vi "RPI2 Enable I2C.vi"(8 "Error In":errorcluster, 11 "Install LV Data":T1={"SSH Session"=refnum, "Status Log"="", "Detailed Log"="", "Credentials"={"Hostname or IP"="192.168.7.2", "Username"="root", "Password"=""}, "Target Info"={"OS Version"="", "CPU"="", "Systemd Version"="", "Internet Access"=FALSE, "Device Type"="", "LV Installed Ver"="", "LV Available Ver"="", "LV Upgrade Available"=FALSE, "Hostname"="", "NIC Info"=[]}, "Reboot Required?"=FALSE}) -> (0 "Error Out":errorcluster, 1 "Log":string, 3 "Install LV Data":T1={"SSH Session"=refnum, "Status Log"="", "Detailed Log"="", "Credentials"={"Hostname or IP"="192.168.7.2", "Username"="root", "Password"=""}, "Target Info"={"OS Version"="", "CPU"="", "Systemd Version"="", "Internet Access"=FALSE, "Device Type"="", "LV Installed Ver"="", "LV Available Ver"="", "LV Upgrade Available"=FALSE, "Hostname"="", "NIC Info"=[]}, "Reboot Required?"=FALSE})   [LabVIEW 2019, in "LMH-LINX.lvlib"]
uses:
  <vilib>/MakerHub/LINX/LMH-LINX.lvlib
  <vilib>/MakerHub/LINX/Private/Utilties/Target Management/Install LV Data.ctl
  <vilib>/MakerHub/LINX/Private/Utilties/Target Management/Target Info.ctl
  <vilib>/MakerHub/LINX/Private/Utilties/Target Management/NIC Info.ctl
  <vilib>/MakerHub/LINX/Private/Utilties/Target Management/NIC Mode.ctl
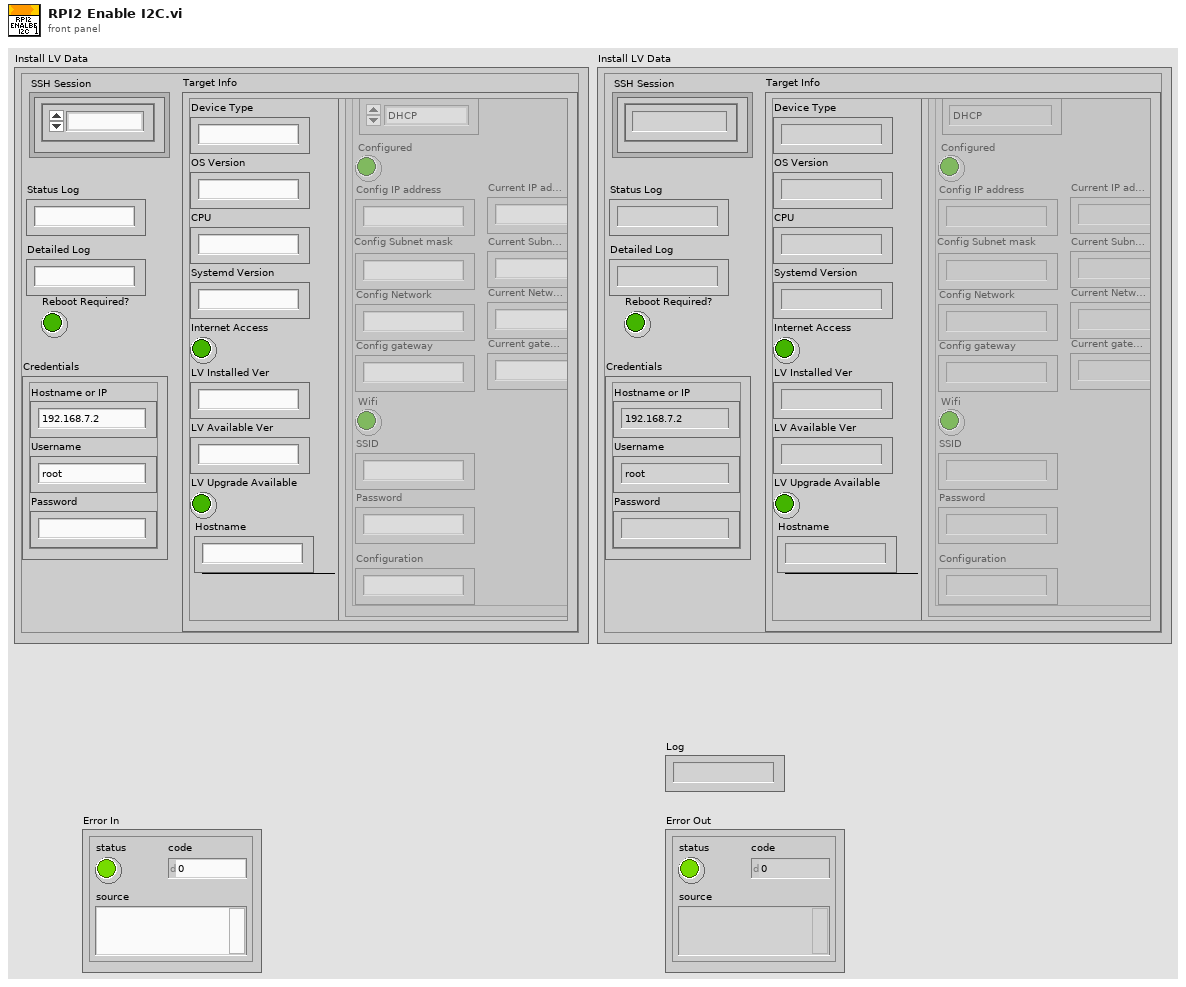
[diagram p1: front panel]
types:
  T1 = typedef "LMH-LINX.lvlib/Install LV Data.ctl" = cluster{"SSH Session":refnum<k1>, "Status Log":string, "Detailed Log":string, "Credentials":cluster{"Hostname or IP":string, "Username":string, "Password":string}, "Target Info":T2, "Reboot Required?":bool}
  T2 = typedef "LMH-LINX.lvlib/Target Info.ctl" = cluster{"OS Version":string, "CPU":string, "Systemd Version":string, "Internet Access":bool, "Device Type":string, "LV Installed Ver":string, "LV Available Ver":string, "LV Upgrade Available":bool, "Hostname":string, "NIC Info":T3[]}
  T3 = typedef "LMH-LINX.lvlib/NIC Info.ctl" = cluster{"Name":string, "NIC Mode":T4, "Configured":bool, "Config IP address":string, "Config Subnet mask":string, "Config Network":string, "Config gateway":string, "Wifi":bool, "SSID":string, "Password":string, "Configuration":string, "Current IP address":string, "Current Subnet mask":string, "Current gateway":string, "Current Network":string}
  T4 = typedef "LMH-LINX.lvlib/NIC Mode.ctl" = enum16{"DHCP", "Static", "Loopback"}
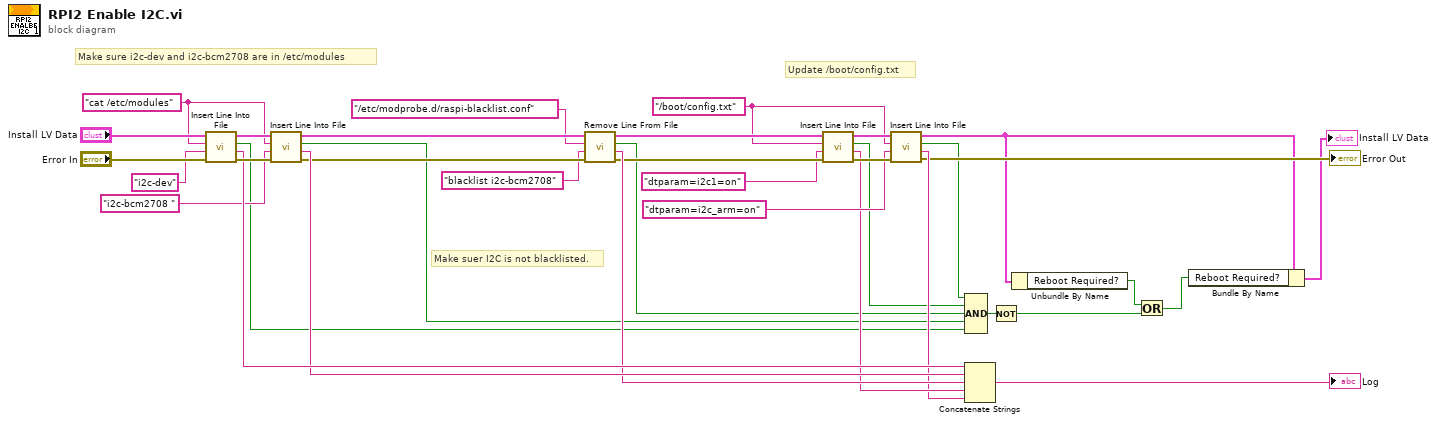
[diagram p0: block diagram]
diagram:
  w15 = "/boot/config.txt"
  w27 = "cat /etc/modules" ("File Path")
  # "Update /boot/config.txt"
  # "Make suer I2C is not blacklisted."
  # "Make sure i2c-dev and i2c-bcm2708 are in /etc/modules"
  n1 = call <vilib>:"Insert Line Into File.vi"("Error In"="Error In", "Line"="i2c-dev" ("File Path"), "File Path"=w27, "Install LV Data"="Install LV Data") -> ("Error Out"=w33:errorcluster, "Log"=w32:string, "Line Alredy Present?"=w7:bool, "Install LV Data"=w34:T1)  [unwired: 4 in]
  n2 = call <vilib>:"Insert Line Into File.vi"("Error In"=w33, "Line"="i2c-bcm2708 " ("File Path"), "File Path"=w27, "Install LV Data"=w34) -> ("Error Out"=w25:errorcluster, "Log"=w31:string, "Line Alredy Present?"=w8:bool, "Install LV Data"=w26:T1)  [unwired: 4 in]
  n3 = call <vilib>:"Remove Line From File.vi"("Error In"=w25, "Line"="blacklist i2c-bcm2708" ("File Path"), "File Path"="/etc/modprobe.d/raspi-blacklist.conf", "Install LV Data"=w26) -> ("Error Out"=w20:errorcluster, "Log"=w22:string, "Line Previously Present?"=w9:bool, "Install LV Data"=w21:T1)  [unwired: 4 in]
  n4 = call <vilib>:"Insert Line Into File.vi"("Error In"=w20, "Line"="dtparam=i2c1=on", "File Path"=w15, "Install LV Data"=w21) -> ("Error Out"=w17:errorcluster, "Log"=w14:string, "Line Alredy Present?"=w10:bool, "Install LV Data"=w18:T1)  [unwired: 4 in]
  n5 = call <vilib>:"Insert Line Into File.vi"("Error In"=w17, "Line"="dtparam=i2c_arm=on", "File Path"=w15, "Install LV Data"=w18) -> ("Error Out"=→"Error Out":errorcluster, "Log"=w13:string, "Line Alredy Present?"=w11:bool, "Install LV Data"=w4:T1)  [unwired: 4 in]
  n6 = Compound Arithmetic op=AND(w11, w10, w9, w8, w7) -> (w6:bool)
  n7 = Concatenate Strings(w32, w31, w22, w14, w13) -> (→"Log":string)
  n8 = Not(x=w6) -> (.not. x?=w5:bool)
  n9 = Unbundle By Name(w4) -> ("Reboot Required?"=w2:bool)
  n10 = Or(x=w2, y=w5) -> (x .or. y?=w1:bool)
  n11 = Bundle By Name(cluster=w4, "Reboot Required?"=w1) -> (→"Install LV Data":T1)
